vi "CRYSwept sine freq or ampl.vi"(6 "Stimulus setup":string, 8 "Calibration setup":string, 9 "Hardware setup":string, 11 "Signal Path":string) -> (2 "Master":cluster{"freq":dbl, "ampl":dbl, "cycles":dbl}[](array[cluster]) {"cycles" format="%.2f"; "ampl" format="%.2f"; "freq" format="%.2f"})   [LabVIEW 2013]
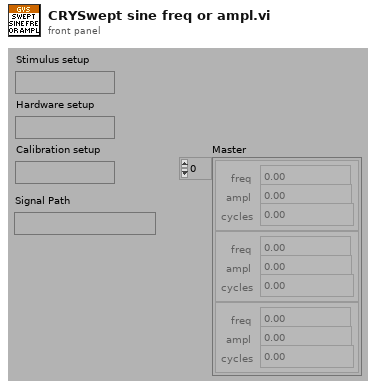
[diagram p1: front panel]
types:
  T1 = typedef "CRYCalibration All Cluster.ctl" = cluster{"Calibration 2D":T2[], "Help":string, "Tab Value":i32, "Input Signal Type":string, "Output Signal Type":string}
  T2 = typedef "CRYCalibration 2DCluster.ctl" = cluster{"Calibration":T3, "Corr Curve":T4, "EQ Curve":T4, "Sens Curve":T4}
  T3 = typedef "CRYCalibration Cluster.ctl" = cluster{"Calibration Step Name":string, "Device":string, "Correction Curve Name":string, "Equalization Curve Name":string, "Sensitivity Curve Name":string, "Corr Folder and File":string, "EQ Folder and File":string, "Sens Folder and File":string, "Corr Step size":u16, "EQ Step size":u16, "Input":bool, "Last Cal Date (sec)":timestamp, "Cha Name":string, "Corr Curve Found":bool, "EQ Curve Found":bool, "Sens Curve Found":bool, "Signal Type":string, "Calibrated Device":string, "Hz":u32}
  T4 = typedef "CRYData Cluster.ctl" = cluster{"Name":string, "Curve":cluster{"x":dbl, "y":dbl, "z":dbl}[], "X data":u16, "Y data":u16, "Z data":u16, "X axis":u16, "Y axis":u16, "Z axis":u16, "X unit":string, "Y unit":string, "Z unit":string, "X dB ref":dbl, "Y dB ref":dbl, "Z dB ref":dbl, "single val":bool, "protected":bool, "display X":bool, "display Y":bool, "display Z":bool, "Test Info":string, "Step No.":i32, "Plot Settings":cluster{"Color":u32, "Interpolation":u8, "Point Style":u8, "Line Style":u8, "Point Color":u32, "Line Width":u8, "Bar Plot Style":u8, "Fill To":i16}, "AutoProtect":bool}
  T5 = typedef "CRYStimulus Parameter.ctl" = cluster{"Name":string, "Level Out":dbl, "Start Freq":dbl, "Stop Freq":dbl, "Steps":u32, "Cycles":u32, "Sweep type":i32, "Freq":dbl, "Start ampl":dbl, "Stop ampl":dbl, "sine waves":cluster{"freq":dbl, "ampl":dbl, "cycles":dbl}[], "wav path":string, "Sweep time":dbl, "Resolution":u16, "Tone type6":u16, "fix/ratio6":u16, "Ratio6":u16, "Difference6":u32, "RatioFreq6":u32}
  T6 = typedef "CRYHardware Channel Info.ctl" = cluster{"ID":i32, "Name":string, "Digital":bool, "Input":bool, "Device Name":string, "Hardware Ch ID":u8, "Vmax (V)":dbl, "Latency (samples)":dbl, "Sampling Rate (Hz)":u32, "Bit Depth":u32, "Anti-aliasing Factor (%fs)":sgl, "DAQmx Channel":tag, "term config":i32, "Coupling":i32, "IEPE en":bool, "ASIOChannel Name":string, "Audio Driver":u16, "ASIOChannel Index":u8}
  T7 = cluster{"Stop Freq Out":dbl, "Level Out":dbl, "Cout":dbl}[]
  T8 = cluster{"Start Freq Out":dbl, "Level Out":dbl, "Bundle Element":dbl}
  T9 = cluster{"Stop Freq Out":dbl, "Level Out":dbl, "Bundle Element":dbl}
  T10 = cluster{"Stop Freq Out":dbl, "Level Out":dbl, "Bundle Element":dbl}[]
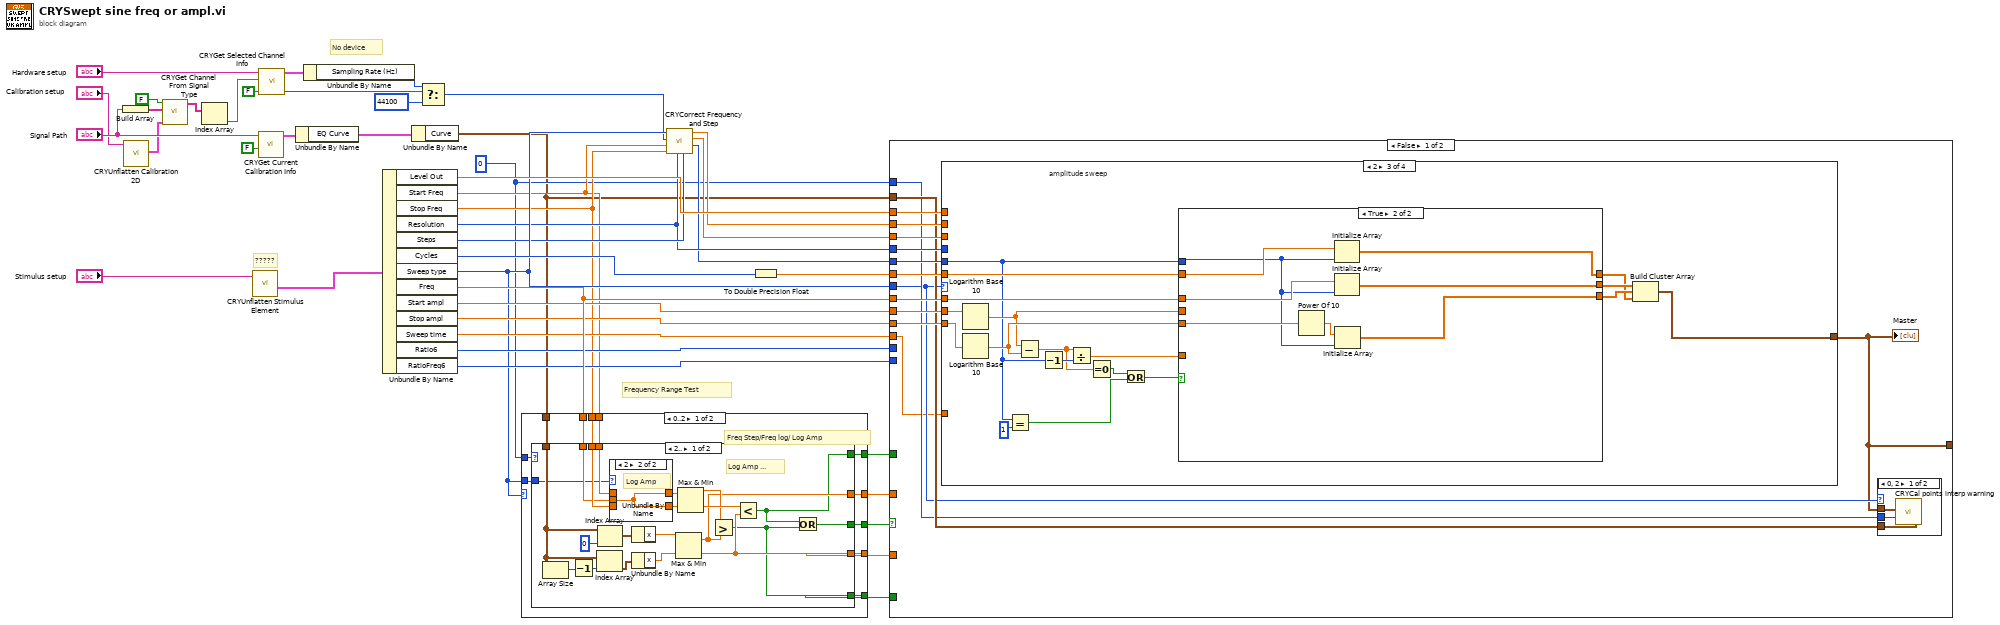
[diagram p0: block diagram]
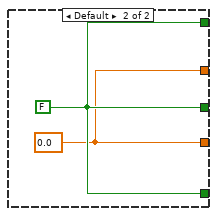
[diagram p3: hidden frame]
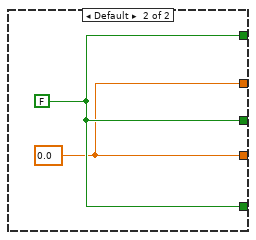
[diagram p4: hidden frame]
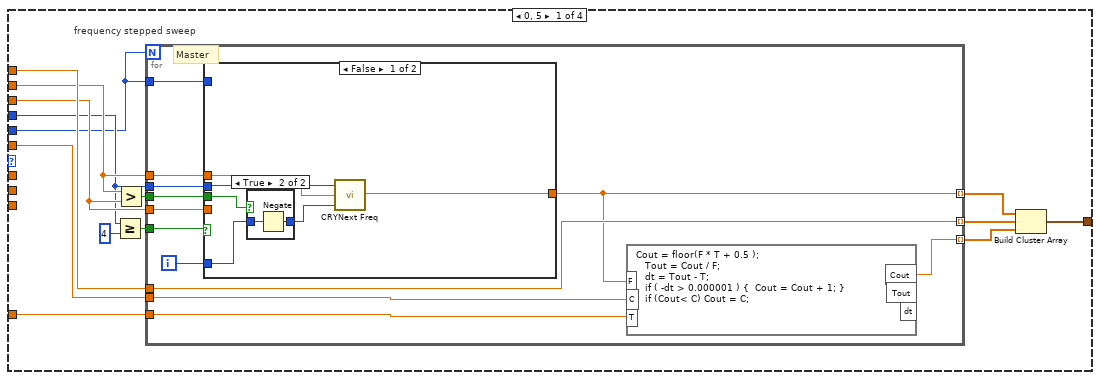
[diagram p6: hidden frame]
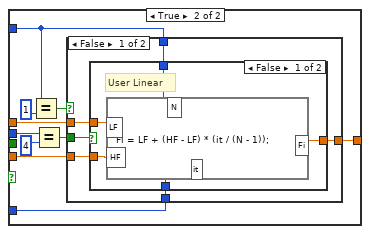
[diagram p8: hidden frame]
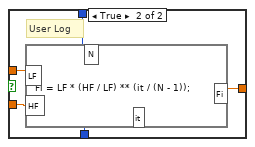
[diagram p9: hidden frame]
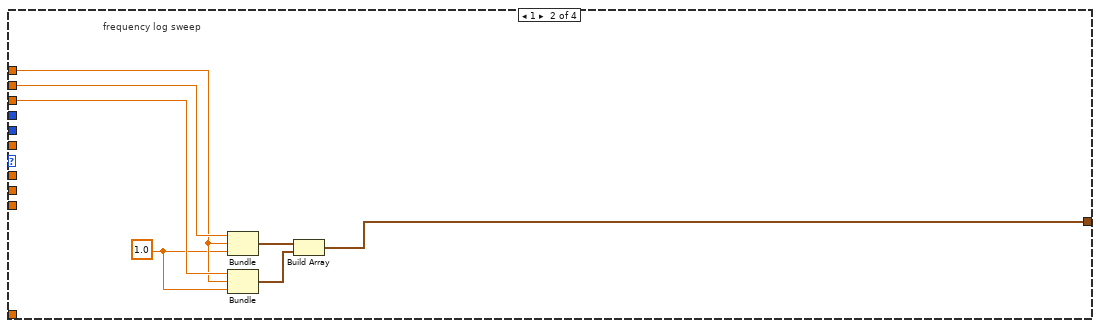
[diagram p11: hidden frame]
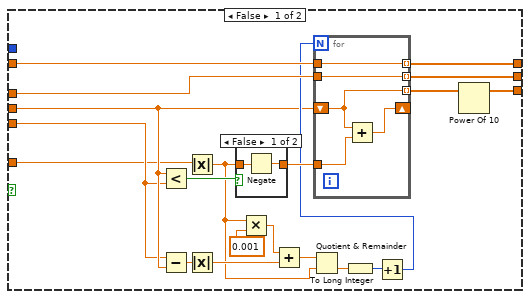
[diagram p12: hidden frame]
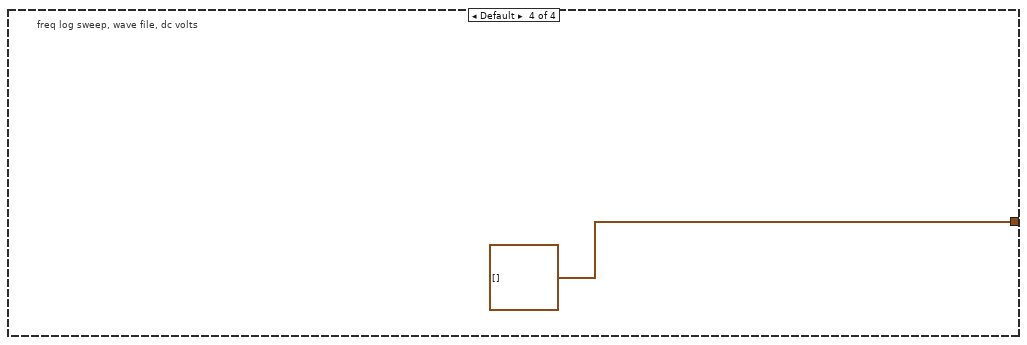
[diagram p14: hidden frame]
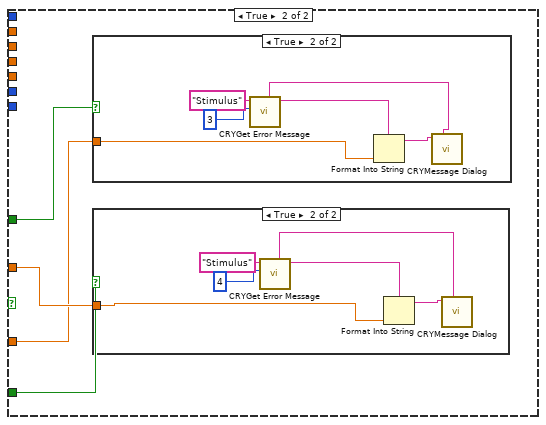
[diagram p15: hidden frame]
diagram:
  w18 = u16 0 ("Device Out")
  # "No device"
  # "?????"
  # "Frequency Range Test"
  n1 = Build Array("Signal Path") -> (w7:string[])
  n2 = call "CRYUnflatten Calibration 2D.vi"("Flattened Calibration"="Calibration setup") -> ("Calibration Step Out"=w2:T1)  [unwired: 8 in, 2 out]
  n3 = call "CRYGet Channel From Signal Type.vi"("Calibration"=w2, "Signal Type Name Array In"=w7, "In/Out?"=FALSE) -> ("Channel Name Array Out"=w6:string[])  [unwired: 7 in, 1 out]
  n4 = Index Array(array=w6) -> (element=w5:string)  [unwired: 1 in]
  n5 = call "CRYUnflatten Stimulus Element.vi"("Unflatten Stimulus Element setup"="Stimulus setup") -> ("Stimulus Para"=w19:T5)  [unwired: 1 in, 9 out]
  n6 = call "CRYGet Current Calibration Info.vi"("Is Input?"=FALSE, "Signal Type Name"="Signal Path") -> ("Calibration All Cluster"=w14:T2)  [unwired: 9 out]
  n7 = call "CRYGet Selected Channel Info.vi"("In/out?"=FALSE, "Channel Name"=w5, "Flattened Hardware"="Hardware setup") -> ("exist?"=w13:bool, "Channel infor"=w23:T6)  [unwired: 7 out]
  n8 = Unbundle By Name(w14) -> ("EQ Curve"=w16:T4)
  n9 = Unbundle By Name(w23) -> ("Sampling Rate (Hz)"=w12:u32)
  n10 = Unbundle By Name(w19) -> ("Level Out"=w38:dbl, "Start Freq"=w25:dbl, "Stop Freq"=w26:dbl, "Resolution"=w27:u16, "Steps"=w28:u32, "Cycles"=w37:u32, "Sweep type"=w29:i32, "Freq"=w36:dbl, "Start ampl"=w35:dbl, "Stop ampl"=w34:dbl, "Sweep time"=w32:dbl, "Ratio6"=w31:u16, "RatioFreq6"=w30:u32)
  n11 = Unbundle By Name(w16) -> ("Curve"=w15:cluster{"x":dbl, "y":dbl, "z":dbl}[])
  n12 = Select(t=w12, s=w13, f=u32 44100) -> (s? t:f=w10:u32)
  n13 = case shown="0..2" w29 {
    tunnel: [w54 w82] -> w43
    tunnel: [w53 w81] -> w42
    tunnel: [w52 w81] -> w41
    tunnel: [w51 w82] -> w40
    tunnel: [w50 w82] -> w39
    tunnel: w25 -> [w49 _]
    tunnel: w26 -> [w48 _]
    tunnel: w36 -> [w47 _]
    tunnel: w18 -> [w46 _]
    tunnel: w15 -> [w45 _]
    tunnel: w29 -> [w44 _]
    frame 0..2 {
      # "Freq Step/Freq log/ Log Amp"
      n14 = case shown="2.." w46 {
        tunnel: w45 -> [w66 _]
        tunnel: w49 -> [w65 _]
        tunnel: w48 -> [w63 _]
        tunnel: w47 -> [w61 _]
        tunnel: [w60 w80] -> w54
        tunnel: [w59 w79] -> w53
        tunnel: [w58 w79] -> w52
        tunnel: [w57 w80] -> w51
        tunnel: [w56 w80] -> w50
        tunnel: w44 -> [w55 _]
        frame 2.. {
          # "Log Amp ..."
          n15 = Array Size(array=w66) -> (size(s)=w68:i32)
          n16 = Decrement(x=w68) -> (x-1=w67:i32)
          n17 = Index Array(array=w66, index=w67) -> (element=w73:cluster{"x":dbl, "y":dbl, "z":dbl})
          n18 = Index Array(array=w66, index=0) -> (element=w72:cluster{"x":dbl, "y":dbl, "z":dbl})
          n19 = case shown="2" w55 {
            tunnel: [w77 w78] -> w64
            tunnel: w65 -> [w77 _]
            tunnel: [w76 w78] -> w62
            tunnel: w63 -> [w76 _]
            tunnel: w61 -> [_ w78]
            frame Default {
            }
            frame 2 {
              # "Log Amp"
            }
          }
          n20 = Unbundle By Name(w72) -> ("x"=w71:dbl)
          n21 = Unbundle By Name(w73) -> ("x"=w70:dbl)
          n22 = Max & Min(x=w71, y=w70) -> (max(x,y)=w59:dbl, min(x,y)=w58:dbl)
          n23 = Max & Min(x=w64, y=w62) -> (max(x,y)=w74:dbl, min(x,y)=w75:dbl)
          n24 = Greater?(x=w74, y=w59) -> (0:w56:bool)
          n25 = Less?(x=w75, y=w58) -> (x < y?=w57:bool)
          n26 = Or(x=w57, y=w56) -> (x .or. y?=w60:bool)
        }
        frame Default {
          w79 = 0.0 ("Hz")
          w80 = FALSE
        }
      }
    }
    frame Default {
      w81 = 0.0 ("Hz")
      w82 = FALSE
    }
  }
  n27 = call "CRYCorrect Frequency and Step.vi"("Steps"=w28, "Resolution"=w27, "Stop Frequency"=w26, "Start Frequency"=w25, "Sampling Rate"=w10, "Sweep type"=w29) -> ("Steps"=w22:u32, "Stop Freq Out"=w20:dbl, "Start Freq Out"=w21:dbl)  [unwired: 3 in]
  n28 = To Double Precision Float(number=w37) -> (double precision float=w33:dbl)
  n29 = case shown="False" w43 {
    tunnel: w42 -> [_ w227]
    tunnel: w41 -> [_ w226]
    tunnel: w40 -> [_ w225]
    tunnel: w39 -> [_ w224]
    tunnel: w27 -> [w96 _]
    tunnel: w21 -> [w95 _]
    tunnel: w20 -> [w94 _]
    tunnel: w38 -> [w93 _]
    tunnel: w22 -> [w92 _]
    tunnel: w33 -> [w91 _]
    tunnel: w29 -> [w85 _]
    tunnel: w36 -> [w90 _]
    tunnel: w35 -> [w89 _]
    tunnel: w34 -> [w88 _]
    tunnel: w15 -> [w87 _]
    tunnel: w18 -> [w86 _]
    tunnel: w32 -> [w84 _]
    tunnel: w31 -> [_ _]
    tunnel: w30 -> [_ _]
    tunnel: [w83 _] -> _
    frame False {
      n30 = case shown="2" w85 {
        tunnel: w96 -> [w106 _ _ _]
        tunnel: w95 -> [w107 w165 _ _]
        tunnel: w94 -> [w109 w164 _ _]
        tunnel: w93 -> [w110 w163 _ _]
        tunnel: w92 -> [w105 _ w169 _]
        tunnel: w91 -> [w101 _ w185 _]
        tunnel: w90 -> [_ _ w186 _]
        tunnel: w89 -> [_ _ w177 _]
        tunnel: w88 -> [_ _ w176 _]
        tunnel: [w111 w166 w181 cluster{dbl, "Level Out":dbl, dbl}[] []] -> w83
        tunnel: w84 -> [w100 _ _ _]
        frame 0, 5 {
          # "frequency stepped sweep"
          n31 = Greater Or Equal?(x=w106, y=u16 4) -> (x >= y?=w112:bool)
          n32 = Greater?(x=w107, y=w109) -> (0:w108:bool)
          n33 = for {
            N: w105 -> [_]
            tunnel: w109 -> [w125]
            tunnel: w107 -> [w124]
            tunnel: w112 -> [w123]
            tunnel: w106 -> [w120]
            tunnel: [w114] -> w104 mode=indexing
            tunnel: w108 -> [w122]
            tunnel: [w115] -> w102 mode=indexing
            tunnel: [w119] -> w103 mode=indexing
            tunnel: w110 -> [w119]
            tunnel: w101 -> [w116]
            tunnel: w105 -> [w121]
            tunnel: w100 -> [w117]
            i -> [w118]
            # "Master"
            n34 = case shown="False" w123 {
              tunnel: [w130 w144] -> w114
              tunnel: w124 -> [w128 w143]
              tunnel: w125 -> [_ w142]
              tunnel: w120 -> [w129 w137]
              tunnel: w122 -> [w127 _]
              tunnel: w121 -> [_ w139]
              tunnel: w118 -> [w126 w138]
              frame False {
                n35 = case shown="True" w127 {
                  tunnel: w126 -> [w132 w134]
                  tunnel: [w132 w133] -> w131
                  frame False {
                  }
                  frame True {
                    n36 = Negate(x=w134) -> (-x=w133:i32)
                  }
                }
                n37 = call "CRYNext Freq.vi"("No. Steps"=w131, "Freq In"=w128, "Step size"=w129) -> ("Next Freq"=w130:dbl)  [unwired: 2 out]
              }
              frame True {
                n38 = Equal?(x=w139, y=u32 1) -> (x = y?=w141:bool)
                n39 = Equal?(x=w137, y=u16 4) -> (x = y?=w136:bool)
                n40 = case shown="False" w141 {
                  tunnel: w142 -> [w150 w161]
                  tunnel: w139 -> [w149 _]
                  tunnel: w143 -> [w148 _]
                  tunnel: w138 -> [w147 _]
                  tunnel: [w146 w161] -> w144
                  tunnel: w136 -> [w145 _]
                  frame False {
                    n41 = case shown="False" w145 {
                      tunnel: w150 -> [w155 w160]
                      tunnel: w149 -> [w154 w159]
                      tunnel: w148 -> [w153 w158]
                      tunnel: w147 -> [w152 w157]
                      tunnel: [w151 w156] -> w146
                      frame False {
                        # "User Linear"
                        n42 = formula code="Fi = LF + (HF - LF) * (it / (N - 1));"("HF"=w155, "LF"=w153, "N"=w154, "it"=w152) -> ("Fi"=w151:dbl)
                      }
                      frame True {
                        # "User Log"
                        n43 = formula code="Fi = LF * (HF / LF) ** (it / (N - 1));"("HF"=w160, "LF"=w158, "N"=w159, "it"=w157) -> ("Fi"=w156:dbl)
                      }
                    }
                  }
                  frame True {
                  }
                }
              }
            }
            n44 = formula code="Cout = floor(F * T + 0.5 );\n   Tout = Cout / F;\n   dt = Tout - T;\n   if ( -dt > 0.000001 ) {  Cout = Cout + 1; }\n   if (Cout< C) Cout = C;"("F"=w114, "T"=w117, "C"=w116) -> ("Cout"=w115:dbl)  [unwired: 2 out]
          }
          n45 = Build Cluster Array(w104, w103, w102) -> (w111:T7)
        }
        frame 1 {
          w162 = 1.0 ("Bundle Element")
          # "frequency log sweep"
          n46 = Bundle("Start Freq Out"=w165, "Level Out"=w163, "Bundle Element"=w162) -> (w168:T8)  [unwired: 1 out]
          n47 = Bundle("Stop Freq Out"=w164, "Level Out"=w163, "Bundle Element"=w162) -> (w167:T9)  [unwired: 1 out]
          n48 = Build Array(w168, w167) -> (w166:T10)
        }
        frame 2 {
          # "amplitude sweep"
          n49 = Logarithm Base 10(1:w177) -> (0:w174:dbl)
          n50 = Logarithm Base 10(1:w176) -> (0:w175:dbl)
          n51 = Equal?(x=w169, y=u32 1) -> (x = y?=w171:bool)
          n52 = Subtract(x=w174, y=w175) -> (x-y=w172:dbl)
          n53 = Decrement(x=w169) -> (x-1=w179:u32)
          n54 = Divide(x=w172, y=w179) -> (x/y=w173:dbl)
          n55 = Equal To 0?(x=w172) -> (x = 0?=w178:bool)
          n56 = Or(x=w178, y=w171) -> (x .or. y?=w170:bool)
          n57 = case shown="True" w170 {
            tunnel: w175 -> [w190 w222]
            tunnel: w174 -> [w191 _]
            tunnel: w186 -> [w198 w219]
            tunnel: w185 -> [w197 w221]
            tunnel: [w196 w218] -> w184
            tunnel: [w187 w216] -> w183
            tunnel: [w195 w220] -> w182
            tunnel: w173 -> [w189 _]
            tunnel: w169 -> [_ w215]
            frame False {
              n58 = Less?(x=w191, y=w190) -> (x < y?=w206:bool)
              n59 = Subtract(x=w190, y=w191) -> (x-y=w205:dbl)
              n60 = Absolute Value(x=w189) -> (abs(x)=w200:dbl)
              n61 = Absolute Value(x=w205) -> (abs(x)=w202:dbl)
              n62 = case shown="False" w206 {
                tunnel: w200 -> [w213 w214]
                tunnel: [w212 w214] -> w199
                frame False {
                  n63 = Negate(x=w213) -> (-x=w212:dbl)
                }
                frame True {
                }
              }
              n64 = Multiply(x=w200, y=0.001) -> (x*y=w203:dbl)
              n65 = Add(x=w203, y=w202) -> (x+y=w201:dbl)
              n66 = Quotient & Remainder(x=w201, y=w200) -> (floor(x/y)=w194:dbl)  [unwired: 1 out]
              n67 = To Long Integer(number=w194) -> (32bit integer=w193:i32)
              n68 = Increment(x=w193) -> (x+1=w192:i32)
              n69 = for {
                N: w192 -> [_]
                shift-right: [w210] -> _
                shift-left: w191 -> [w209]
                tunnel: w199 -> [w211]
                tunnel: [w209] -> w188 mode=indexing
                tunnel: w198 -> [w208]
                tunnel: w197 -> [w207]
                tunnel: [w208] -> w196 mode=indexing
                tunnel: [w207] -> w195 mode=indexing
                n70 = Add(x=w209, y=w211) -> (x+y=w210:dbl)
              }
              n71 = Power Of 10(x=w188) -> (10^x=w187:dbl[])
            }
            frame True {
              n72 = Power Of 10(x=w222) -> (10^x=w217:dbl)
              n73 = Initialize Array(w221, w215) -> (w220:dbl[])
              n74 = Initialize Array(w219, w215) -> (w218:dbl[])
              n75 = Initialize Array(w217, w215) -> (w216:dbl[])
            }
          }
          n76 = Build Cluster Array(w184, w183, w182) -> (w181:cluster{"Freq":dbl, dbl, dbl}[])
        }
        frame Default {
          # "freq log sweep, wave file, dc volts"
        }
      }
      "Master" <- w83
      n77 = case shown="0, 2" w85 {
        tunnel: w83 -> [w99 _]
        tunnel: w87 -> [w98 _]
        tunnel: w86 -> [w97 _]
        frame 0, 2 {
          n78 = call "CRYCal points interp warning.vi"("Device"=w97, "Sine waves"=w99, "Equalization"=w98) -> ()  [unwired: 9 out]
        }
        frame Default {
        }
      }
    }
    frame True {
      n79 = case shown="True" w225 {
        tunnel: w226 -> [_ w233]
        frame False {
        }
        frame True {
          n80 = call "CRYGet Error Message.vi"("Error No"=3, "Kind"="Stimulus") -> ("Message"=w230:string, "Window Title"=w228:string)  [unwired: 4 in, 4 out]
          n81 = Format Into String(format string=w230, w233) -> (resulting string=w229:string)  [unwired: 2 in, 1 out]
          n82 = call "CRYMessage Dialog.vi"("Window Title"=w228, "Message Content"=w229) -> ()  [unwired: 8 in, 2 out]
        }
      }
      n83 = case shown="True" w224 {
        tunnel: w227 -> [_ w237]
        frame False {
        }
        frame True {
          n84 = call "CRYGet Error Message.vi"("Error No"=4, "Kind"="Stimulus") -> ("Message"=w236:string, "Window Title"=w234:string)  [unwired: 4 in, 4 out]
          n85 = Format Into String(format string=w236, w237) -> (resulting string=w235:string)  [unwired: 2 in, 1 out]
          n86 = call "CRYMessage Dialog.vi"("Window Title"=w234, "Message Content"=w235) -> ()  [unwired: 8 in, 2 out]
        }
      }
    }
  }
